vi "Format Bead String (SubVI).vi"(7 "Bead #":i32, 10 "Moves":dbl[](array[numeric]), 11 "Triggers":cluster{dbl[], dbl[]}[](array[cluster])) -> (3 "Bead String":string)   [LabVIEW 2016]
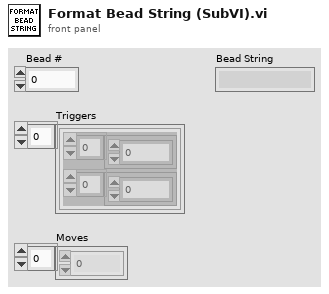
[diagram p1: front panel]
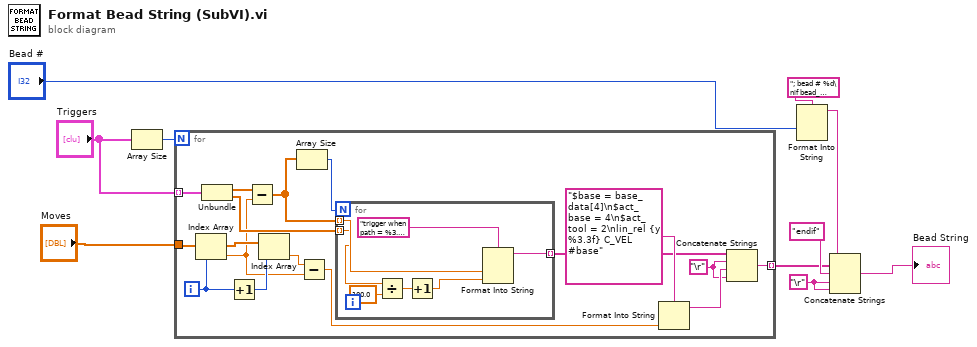
[diagram p0: block diagram]
diagram:
  w1 = "\r"
  n1 = Array Size(array="Triggers") -> (size(s)=w2:i32)
  n2 = for {
    N: w2 -> [_]
    tunnel: "Moves" -> [w22]
    tunnel: "Triggers" -> [w26] mode=indexing
    tunnel: [w11] -> w7 mode=indexing
    i -> [w24]
    w12 = "\r"
    n3 = Index Array(array=w22, index=w24) -> (element=w18:dbl)
    n4 = Unbundle(w26) -> (w25:dbl[], w20:dbl[])
    n5 = Increment(x=w24) -> (x+1=w23:i32)
    n6 = Subtract(x=w25, y=w18) -> (x-y=w17:dbl[])
    n7 = Index Array(array=w22, index=w23) -> (element=w19:dbl)
    n8 = Array Size(array=w17) -> (size(s)=w21:i32)
    n9 = Subtract(x=w19, y=w18) -> (x-y=w15:dbl)
    n10 = for {
      N: w21 -> [_]
      tunnel: w20 -> [w30] mode=indexing
      tunnel: [w32] -> w14 mode=indexing
      tunnel: w17 -> [w31] mode=indexing
      n11 = Divide(x=w30, y=100.0) -> (x/y=w28:dbl)
      n12 = Increment(x=w28) -> (x+1=w27:dbl)
      n13 = Format Into String(format string="trigger when path = %3.3f ONSTART delay = 0 DO $anout[27] = wr_speed*%3.3f\n", w31, w27) -> (resulting string=w32:string)  [unwired: 2 in, 1 out]
    }
    n14 = Format Into String(format string="$base = base_data[4]\n$act_base = 4\n$act_tool = 2\nlin_rel {y  %3.3f} C_VEL #base", w15) -> (resulting string=w13:string)  [unwired: 2 in, 1 out]
    n15 = Concatenate Strings(w14, w12, w13, w12) -> (w11:string)
  }
  n16 = Format Into String(format string="; bead # %d\nif bead_order[j] == %d then \n\n", "Bead #", "Bead #") -> (resulting string=w8:string)  [unwired: 2 in, 1 out]
  n17 = Concatenate Strings(w8, w7, "endif", w1, w1) -> (→"Bead String":string)
